vi "MergeASCArray.vi"(1 "Array2":dbl[](array[numeric]), 2 "Array1":dbl[](array[numeric])) -> (0 "Merged Array":dbl[](array[numeric]))   [LabVIEW 2016]
panel:
  # "Usage :  Merge 2 array Array1、Array2  ( must be  sorted by ASC  already) by ASC sort order. If element is equal,then merge to  one."
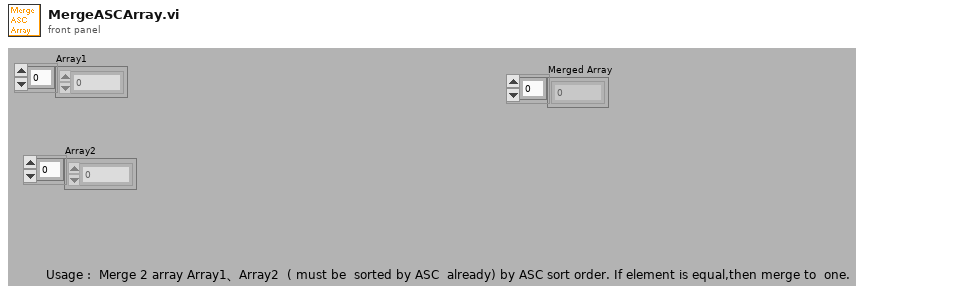
[diagram p1: front panel]
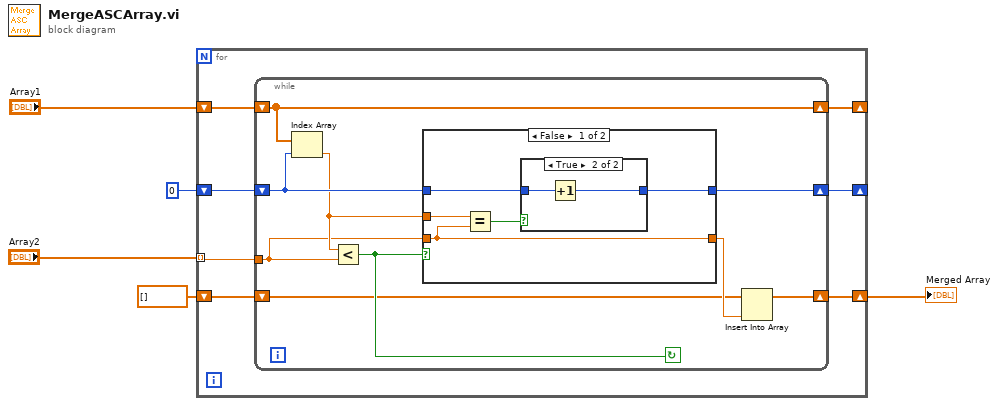
[diagram p0: block diagram]
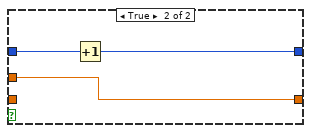
[diagram p3: hidden frame]
diagram:
  n1 = for {
    tunnel: "Array2" -> [w11] mode=indexing
    shift-right: [w9] -> _
    shift-left: "Array1" -> [w12]
    shift-right: [w10] -> _
    shift-left: 0 ("索引") -> [w6]
    shift-right: [w8] -> w1
    shift-left: dbl[] [] -> [w7]
    n2 = while {
      tunnel: w11 -> [w14]
      shift-right: [w16] -> w10
      shift-left: w6 -> [w17]
      shift-right: [w13] -> w9
      shift-left: w12 -> [w13]
      shift-right: [w18] -> w8
      shift-left: w7 -> [w19]
      stop <- w21 continue-if-true
      n3 = Index Array(array=w13, index=w17) -> (element=w15:dbl)
      n4 = Less?(x=w15, y=w14) -> (x < y?=w21:bool)
      n5 = case shown="False" w21 {
        tunnel: w15 -> [w26 w30]
        tunnel: w14 -> [w25 _]
        tunnel: [w25 w30] -> w20
        tunnel: w17 -> [w23 w32]
        tunnel: [w22 w31] -> w16
        frame False {
          n6 = Equal?(x=w26, y=w25) -> (x = y?=w24:bool)
          n7 = case shown="True" w24 {
            tunnel: w23 -> [w27 w29]
            tunnel: [w27 w28] -> w22
            frame False {
            }
            frame True {
              n8 = Increment(x=w29) -> (x+1=w28:i32)
            }
          }
        }
        frame True {
          n9 = Increment(x=w32) -> (x+1=w31:i32)
        }
      }
      n10 = Insert Into Array(array=w19, new element=w20) -> (w18:dbl[])  [unwired: 1 in]
    }
  }
  "Merged Array" <- w1
